vi "APLUS Reset WH Coil.vi"(8 "Error In":errorcluster, 10 "Reset WattHours":bool, 11 "Modbus Master in":refnum<class "Modbus Master.lvclass">) -> (0 "Error Out":errorcluster, 3 "Modbus Master out":refnum<class "Modbus Master.lvclass">)   [LabVIEW 2018]
uses:
  <vilib>/NI/Modbus Library/API/Master/Modbus Master.lvclass
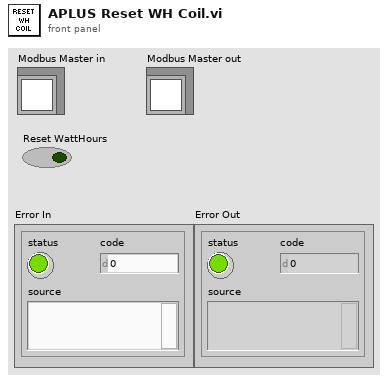
[diagram p1: front panel]
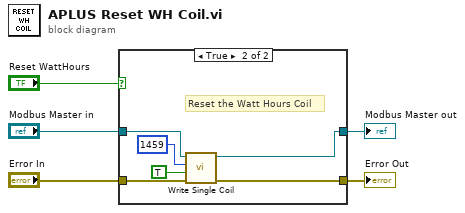
[diagram p0: block diagram]
diagram:
  n1 = case shown="True" "Reset WattHours" {
    tunnel: "Modbus Master in" -> [w7 w12]
    tunnel: [w7 w10] -> w5
    tunnel: "Error In" -> [w6 w9]
    tunnel: [w6 w8] -> w1
    frame False {
    }
    frame True {
      # "Reset the Watt Hours Coil"
      n2 = call-dynamic "Write Single Coil.vi"("error in"=w9, "coil to write"=TRUE ("Coil"), "address"=u16 1459 ("Watt Hour Reset Register"), "Modbus master in"=w12) -> ("error out"=w8:errorcluster, "Modbus master out"=w10:refnum<class "Modbus Master.lvclass">)  [unwired: 6 in]
    }
  }
  "Modbus Master out" <- w5
  "Error Out" <- w1
